vi "Set Window Z-Position.vi"(8 "error in (no error)":errorcluster, 9 "activate? (T)":bool=TRUE, 10 "z-order position":i16(ring) items=["Not Topmost", "Topmost", "Top", "Bottom"], 11 "window refnum":T1) -> (0 "error out":errorcluster, 3 "window refnum out":T1)   [LabVIEW 2020, in "MacroAssert.lvlib" / "WINUTIL.lvlib"]
uses:
  WINUTIL.lvlib
  Window Refnum.ctl
  user32.dll
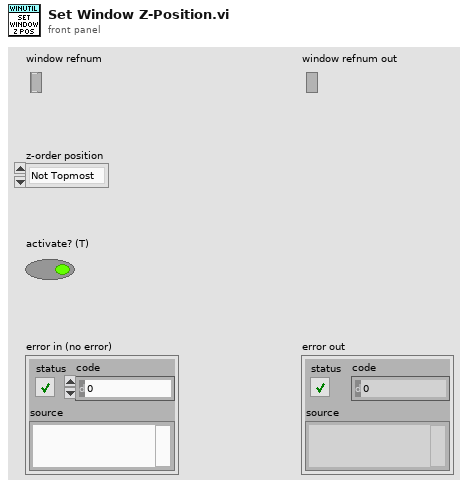
[diagram p1: front panel]
types:
  T1 = typedef "MacroAssert.lvlib/WINUTIL.lvlib/Window Refnum.ctl" = refnum<k1>
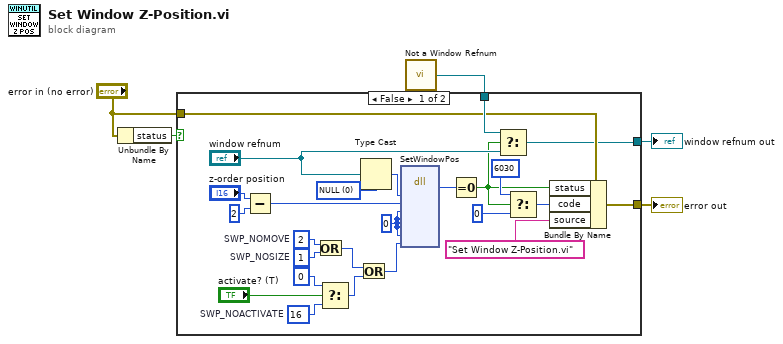
[diagram p0: block diagram]
diagram:
  n1 = Unbundle By Name("error in (no error)") -> ("status"=w4:bool)
  n2 = call "Not a Window Refnum.vi"() -> ("Not a Window Refnum"=w5:T1)
  n3 = case shown="False" w4 {
    tunnel: w5 -> [w15 w31]
    tunnel: "error in (no error)" -> [w8 w32]
    tunnel: [w7 w32] -> w2
    tunnel: [w6 w31] -> w1
    frame False {
      w22 = u32 2  # SWP_NOMOVE
      w23 = u32 1  # SWP_NOSIZE
      w25 = u32 16  # SWP_NOACTIVATE
      w18 = u32 0 items=["NULL"]
      w30 = 0
      n4 = Subtract(x="z-order position", y=i16 2) -> (x-y=w21:i16)
      n5 = Or(x=w22, y=w23) -> (x .or. y?=w28:u32)
      n6 = Select(t=u32 0, s="activate? (T)", f=w25) -> (s? t:f=w27:u32)
      n7 = Or(x=w28, y=w27) -> (x .or. y?=w29:u32)
      n8 = Type Cast(type=w18, x="window refnum") -> (*(type *) &x=w19:u32)
      n9 = dll-call lib="USER32.DLL" fn="SetWindowPos"("hWnd"=w19, "hWndInsertAfter"=w21, "left"=w30, "top"=w30, "width"=w30, "height"=w30, "fuFlags"=w29) -> ("error"=w16:i32)  [unwired: 9 in, 3 out]
      n10 = Equal To 0?(x=w16) -> (x = 0?=w10:bool)
      n11 = Select(t=w15, s=w10, f="window refnum") -> (s? t:f=w6:T1)
      n12 = Select(t=6030, s=w10, f=0) -> (s? t:f=w11:i32)
      n13 = Bundle By Name(cluster=w8, "status"=w10, "code"=w11, "source"="Set Window Z-Position.vi") -> (w7:errorcluster)
    }
    frame True {
    }
  }
  "window refnum out" <- w1
  "error out" <- w2
